vi "ActionVIOnDelete.vi"(6 "All deleted Refs":T1[](array[typedef]) format="%.0x", 8 "error in (no error)":errorcluster, 11 "Item Ref in":T1 format="%.0x") -> (0 "error out":errorcluster, 3 "Item Ref out":T1 format="%.0x")   [LabVIEW 2019, in "Software Multi-Plex System Explorer.lvlib"]
uses:
  Software Multi-Plex System Explorer.lvlib
  <vilib>/NI VeriStand/Custom Device API/Custom Device Item Ref.ctl
  Shared/Constants.vi
  <vilib>/NI VeriStand/Custom Device API/Custom Device API.lvlib
  Shared/Software Multi-Plex Shared.lvlib
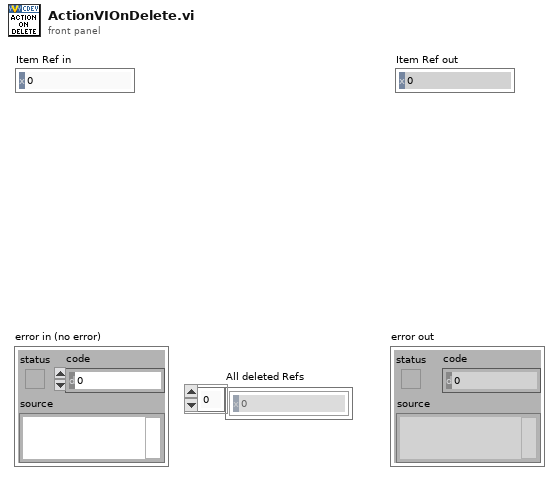
[diagram p1: front panel]
types:
  T1 = typedef "Custom Device API.lvlib/Custom Device Item Ref.ctl" = u64
  T2 = typedef "Custom Device API.lvlib/Custom Device Pointer.ctl" = refnum<k24>
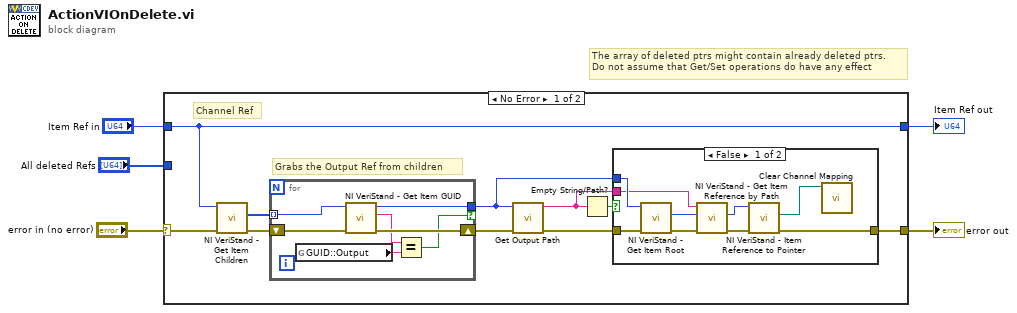
[diagram p0: block diagram]
diagram:
  # "The array of deleted ptrs might contain already deleted ptrs.\nDo not assume that Get/Set operations do have any effect"
  n1 = case shown="No Error" "error in (no error)" {
    selector: "error in (no error)" -> [w11 w34]
    tunnel: [w15 w34] -> w4
    tunnel: "Item Ref in" -> [w9 w33]
    tunnel: [w9 w33] -> w2
    tunnel: "All deleted Refs" -> [_ _]
    frame No Error {
      # "Grabs the Output Ref from children"
      # "Channel Ref"
      n2 = call <vilib>:"NI VeriStand - Get Item Children.vi"("error in (no error)"=w11, "Item Ref in"=w9) -> ("error out"=w10:errorcluster, "Child Refs"=w12:T1[])  [unwired: 6 in, 2 out]
      n3 = for {
        tunnel: [w16] -> w7 if=w19
        tunnel: w12 -> [w22] mode=indexing
        shift-right: [w20] -> w8
        shift-left: w10 -> [w21]
        n4 = global read "Constants.vi" "GUID::Output"() -> (w17:string)
        n5 = call <vilib>:"NI VeriStand - Get Item GUID.vi"("error in (no error)"=w21, "Item Ref in"=w22) -> ("error out"=w20:errorcluster, "GUID"=w18:string, "Item Ref out"=w16:T1)  [unwired: 7 in]
        n6 = Equal?(x=w18, y=w17) -> (x = y?=w19:bool)
      }
      n7 = call "Get Output Path.vi"("error in (no error)"=w8, "Item Ref in"=w7) -> ("error out"=w13:errorcluster, "Output Path"=w6:string)  [unwired: 7 in, 1 out]
      n8 = Empty String/Path?(string/path=w6) -> (empty?=w14:bool)
      n9 = case shown="False" w14 {
        tunnel: w13 -> [w29 w32]
        tunnel: w6 -> [w23 _]
        tunnel: [w30 w32] -> w15
        tunnel: w7 -> [w26 _]
        frame False {
          n10 = call <vilib>:"NI VeriStand - Get Item Root.vi"("error in (no error)"=w29, "Item Ref in"=w26) -> ("error out"=w28:errorcluster, "Root Ref out"=w27:T1)  [unwired: 6 in, 2 out]
          n11 = call <vilib>:"NI VeriStand - Get Item Reference by Path.vi"("error in (no error)"=w28, "Root Ref"=w27, "Item Path in"=w23) -> ("error out"=w31:errorcluster, "Item Ref"=w24:T1)  [unwired: 5 in, 2 out]
          n12 = call <vilib>:"NI VeriStand - Item Reference to Pointer.vi"("error in (no error)"=w31, "Item Ref in"=w24) -> ("error out"=w30:errorcluster, "Node Pointer"=w25:T2)  [unwired: 6 in, 2 out]
          n13 = call "Clear Channel Mapping.vi"("Destination"=w25) -> ()  [unwired: 11 in]
        }
        frame True {
        }
      }
    }
    frame Error {
    }
  }
  "error out" <- w4
  "Item Ref out" <- w2
